vi "Spray_setup.vi"(3 "Temp limit on":bool=TRUE, 4 "Amplitude":dbl, 5 "Lower temp limit":dbl, 6 "Pulse":dbl, 7 "Upper temp limit":dbl, 8 "error in (no error)":errorcluster, 10 "Time limit":dbl, 11 "Time limit on":bool=TRUE) -> (0 "error out":errorcluster)   [LabVIEW 2015]
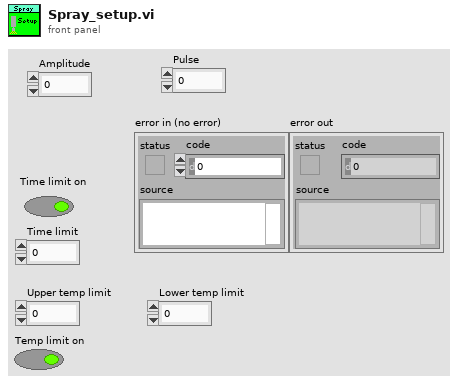
[diagram p1: front panel]
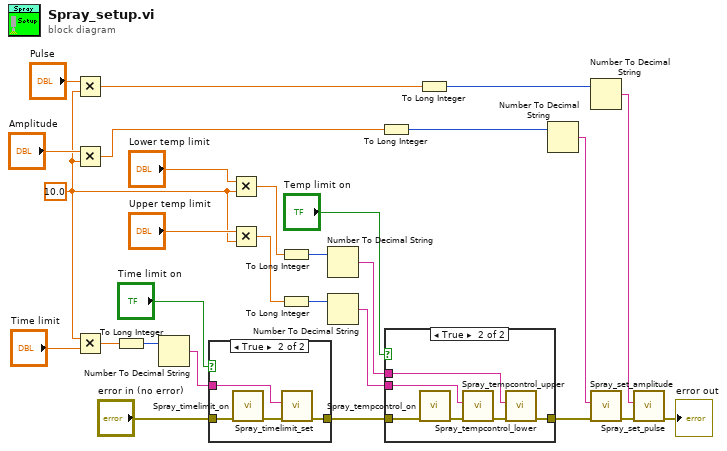
[diagram p0: block diagram]
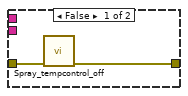
[diagram p2: hidden frame]
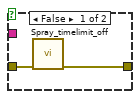
[diagram p3: hidden frame]
diagram:
  w11 = 10.0
  n1 = Multiply(x="Pulse", y=w11) -> (x*y=w8:dbl)
  n2 = Multiply(x="Amplitude", y=w11) -> (x*y=w9:dbl)
  n3 = Multiply(x=w11, y="Time limit") -> (x*y=w2:dbl)
  n4 = To Long Integer(number=w2) -> (32bit integer=w1:i32)
  n5 = Number To Decimal String(number=w1) -> (decimal integer string=w26:string)  [unwired: 1 in]
  n6 = case shown="True" "Time limit on" {
    tunnel: w26 -> [_ w34]
    tunnel: [w30 w32] -> w25
    tunnel: "error in (no error)" -> [w29 w31]
    frame False {
      n7 = call "Spray_timelimit_off.vi"("error in (no error)"=w29) -> ("error out"=w30:errorcluster)  [unwired: 10 in]
    }
    frame True {
      n8 = call "Spray_timelimit_on.vi"("error in (no error)"=w31) -> ("error out"=w33:errorcluster)  [unwired: 10 in]
      n9 = call "Spray_timelimit_set.vi"("error in (no error)"=w33, "input 1"=w34) -> ("error out"=w32:errorcluster)  [unwired: 9 in]
    }
  }
  n10 = Multiply(x="Lower temp limit", y=w11) -> (x*y=w6:dbl)
  n11 = Multiply(x="Upper temp limit", y=w11) -> (x*y=w4:dbl)
  n12 = To Long Integer(number=w6) -> (32bit integer=w5:i32)
  n13 = To Long Integer(number=w4) -> (32bit integer=w3:i32)
  n14 = Number To Decimal String(number=w5) -> (decimal integer string=w23:string)  [unwired: 1 in]
  n15 = Number To Decimal String(number=w3) -> (decimal integer string=w24:string)  [unwired: 1 in]
  n16 = To Long Integer(number=w9) -> (32bit integer=w10:i32)
  n17 = case shown="True" "Temp limit on" {
    tunnel: w25 -> [w36 w42]
    tunnel: w24 -> [_ w39]
    tunnel: w23 -> [_ w38]
    tunnel: [w35 w37] -> w22
    frame False {
      n18 = call "Spray_tempcontrol_off.vi"("error in (no error)"=w36) -> ("error out"=w35:errorcluster)  [unwired: 10 in]
    }
    frame True {
      n19 = call "Spray_tempcontrol_on.vi"("error in (no error)"=w42) -> ("error out"=w41:errorcluster)  [unwired: 10 in]
      n20 = call "Spray_tempcontrol_upper.vi"("error in (no error)"=w41, "input 1"=w39) -> ("error out"=w40:errorcluster)  [unwired: 9 in]
      n21 = call "Spray_tempcontrol_lower.vi"("error in (no error)"=w40, "input 1"=w38) -> ("error out"=w37:errorcluster)  [unwired: 9 in]
    }
  }
  n22 = To Long Integer(number=w8) -> (32bit integer=w7:i32)
  n23 = Number To Decimal String(number=w10) -> (decimal integer string=w18:string)  [unwired: 1 in]
  n24 = Number To Decimal String(number=w7) -> (decimal integer string=w17:string)  [unwired: 1 in]
  n25 = call "Spray_set_amplitude.vi"("input 1"=w18, "error in (no error)"=w22) -> ("error out"=w21:errorcluster)  [unwired: 8 in]
  n26 = call "Spray_set_pulse.vi"("error in (no error)"=w21, "input 1"=w17) -> ("error out"=→"error out":errorcluster)  [unwired: 9 in]
